vi "Event Handler.vi"(8 "error in (no error)":errorcluster, 10 "Stop Event Handler":refnum<user-event>, 11 "SpecificString in":refnum<class "SpecificString.lvclass">) -> (0 "error out":errorcluster)   [LabVIEW 2018, in "SpecificString.lvclass"]
doc: "The <b>Event Handler VI</b> is a dynamic dispatch VI that should be overwritten if events are needed to create the enhanced QControl. \n\nBy inheriting from the main Control.lvclass the overwritten <b>Event Handler VI</b> will be launched asynchronously in the initialization of the QControl.\n<b> </b> <b> </b>\n©2016 Q Software Innovations, LLC (QSI)\nwritten by Quentin Alldredge\nproduced in LabVIEW 2015\n\nsupport@qsoftwareinnovations.com\nwww.qsoftwareinnovations.com\n\nAll rights reserved.\n\nRedistribution and use in source and binary forms, with or without modification, are permitted provided that the following conditions are met:\n\n * Redistributions of source code must retain the above copyright notice, this list of conditions and the following disclaimer.\n * Redistributions in binary form must reproduce the above copyright notice, this list of conditions and the following disclaimer in the documentation and/or other materials provided with the distribution.\n * Neither the name of Q Software Innovations, LLC. nor the names of its contributors may be used to endorse or promote products derived from this software without specific prior written permission.\n\nTHIS SOFTWARE IS PROVIDED BY THE COPYRIGHT HOLDERS AND CONTRIBUTORS \"AS IS\" AND ANY EXPRESS OR IMPLIED WARRANTIES, INCLUDING, BUT NOT LIMITED TO, THE IMPLIED WARRANTIES OF MERCHANTABILITY AND FITNESS FOR A PARTICULAR PURPOSE ARE DISCLAIMED. IN NO EVENT SHALL THE COPYRIGHT OWNER OR CONTRIBUTORS BE LIABLE FOR ANY DIRECT, INDIRECT, INCIDENTAL, SPECIAL, EXEMPLARY, OR CONSEQUENTIAL DAMAGES (INCLUDING, BUT NOT LIMITED TO, PROCUREMENT OF SUBSTITUTE GOODS OR SERVICES; LOSS OF USE, DATA, OR PROFITS; OR BUSINESS INTERRUPTION) HOWEVER CAUSED AND ON ANY THEORY OF LIABILITY, WHETHER IN CONTRACT, STRICT LIABILITY, OR TORT (INCLUDING NEGLIGENCE OR OTHERWISE) ARISING IN ANY WAY OUT OF THE USE OF THIS SOFTWARE, EVEN IF ADVISED OF THE POSSIBILITY OF SUCH DAMAGE."
uses:
  SpecificString.lvclass
  D:/National Instruments/LabVIEW 2018/vi.lib/QSI/QControls/QControl Classes/String/String.lvclass
  SpecificString.lvclass/SpecificString.ctl
  Properties/Get Correct Color.vi
  Properties/Get Error Color.vi
  Properties/Get Format.vi
  <vilib>/regexp/Match Regular Expression.xnode
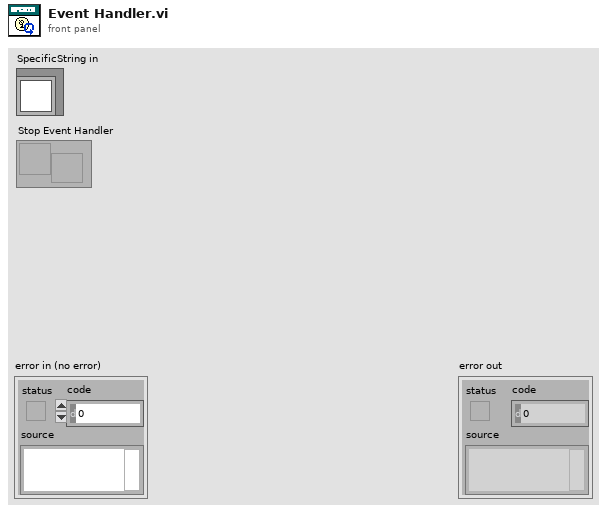
[diagram p1: front panel]
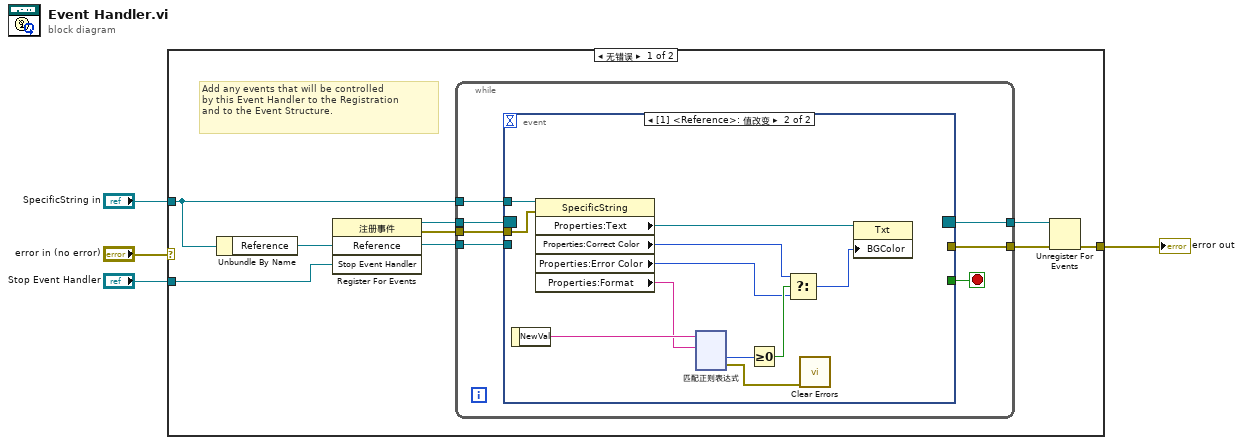
[diagram p0: block diagram]
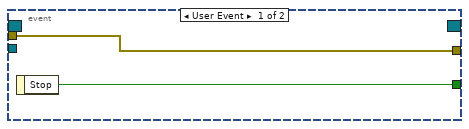
[diagram p2: hidden frame]
diagram:
  n1 = case shown="无错误" "error in (no error)" {
    selector: "error in (no error)" -> [_ w147]
    tunnel: [w9 w147] -> w3
    tunnel: "SpecificString in" -> [w7 _]
    tunnel: "Stop Event Handler" -> [w5 _]
    frame No Error {
      # "Add any events that will be controlled\nby this Event Handler to the Registration\nand to the Event Structure."
      n2 = Unbundle By Name(w7) -> ("Reference"=w6:refnum<vi>)
      n3 = register-events(w6, w5) -> (reference out=w12:refnum<event-registration>, error out=w11:errorcluster)  [unwired: 2 in]
      n4 = while {
        tunnel: w12 -> [w19]
        tunnel: w11 -> [w17]
        tunnel: [w16] -> w10
        tunnel: [w14] -> w8
        tunnel: w6 -> [w13]
        tunnel: w7 -> [w18]
        stop <- w15 stop-if-true
        n5 = event shown="[1] <Reference>: 值改变" {
          selector: w19 -> [_ _]
          dyn-events: [_ _] -> w14
          timeout: _ -> [_ _]
          tunnel: w18 -> [_ w32]
          tunnel: w17 -> [w21 w31]
          tunnel: [w21 _] -> w16
          tunnel: [w20 _] -> w15
          tunnel: w13 -> [_ _]
          event User Event {
            n6 = event-data() -> ("Stop"=w20:bool)  [unwired: 1 in]
          }
          event Value Change {
            n7 = event-data() -> ("NewVal"=w29:string)  [unwired: 1 in]
            n8 = property class="SpecificString"(reference=w32, error in=w31) -> ("Properties:Text"=w30:refnum<vi>, "Properties:Correct Color"=w25:u32, "Properties:Error Color"=w24:u32, "Properties:Format"=w28:string)  [unwired: 2 out]
            n9 = xnode "匹配正则表达式"("输入字符串"=w29, "正则表达式"=w28) -> ("匹配后偏移量"=w27:i32, "错误输出"=w22:errorcluster)  [unwired: 4 in, 3 out]
            n10 = Greater Or Equal To 0?(x=w27) -> (x >= 0?=w26:bool)
            n11 = Select(t=w25, s=w26, f=w24) -> (s? t:f=w23:u32)
            n12 = call <vilib>:"Clear Errors.vi"("error in (no error)"=w22) -> ()  [unwired: 5 in, 2 out]
            n13 = property class="Txt"(reference=w30, "BGColor"=w23) -> ()  [unwired: 1 in, 2 out]
          }
        }
      }
      n14 = Unregister For Events(event registration refnum=w8, error in=w10) -> (error out=w9:errorcluster)
    }
    frame Error {
    }
  }
  "error out" <- w3
